vi "Error Query (Multiple).vi"(0 "VISA Resource Name":refnum<visa-resource-name>, 11 "error in (no error)":errorcluster {"code" format="%.0x"}) -> (4 "VISA Resource Name Out":refnum<visa-resource-name>, 8 "Error":i32[](array[numeric]), 10 "Error Message":string, 15 "error out":errorcluster {"code" format="%.0x"})   [LabVIEW 2012, in "Agilent ESG Series.lvlib"]
doc: "This VI reads the error queue from the instrument. It expects to see errors in SCPI format (#,\"error message\"). It continues to read from the error queue until it reads a 0, \"No error\". If the instrument does not support an error query, a warning is returned."
uses:
  <instrlib>/Agilent ESG Series/Agilent ESG Series.lvlib
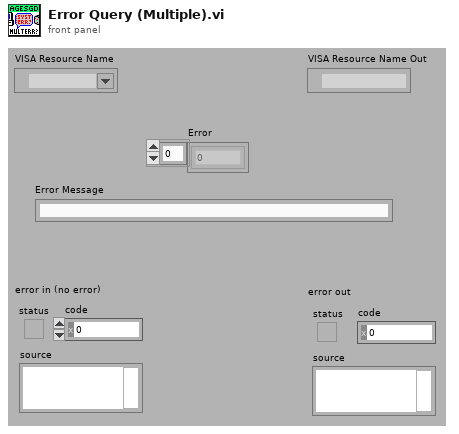
[diagram p1: front panel]
types:
  T1 = cluster{"Status":bool, "Error":i32, "source":string}
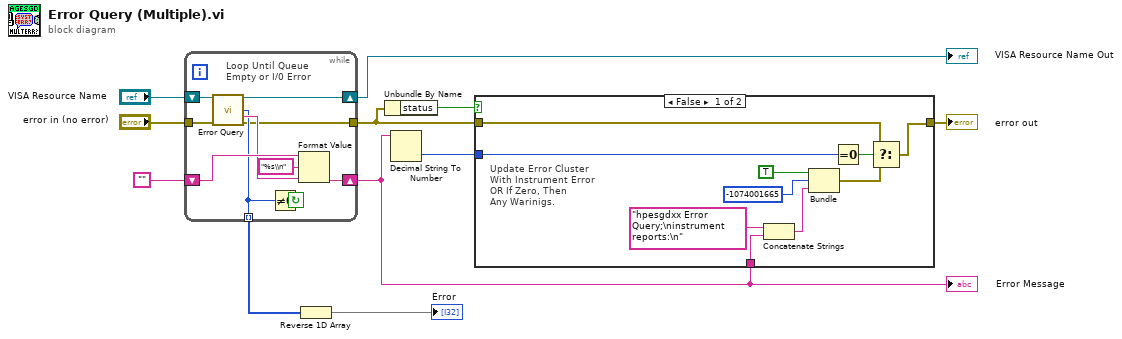
[diagram p0: block diagram]
diagram:
  n1 = while {
    tunnel: "error in (no error)" -> [w12]
    tunnel: [w15] -> w9 mode=indexing
    tunnel: [w13] -> w4
    shift-left: "VISA Resource Name" -> [w14]
    shift-right: [w21] -> w3
    shift-left: "" -> [w18]
    shift-right: [w20] -> w2
    stop <- w16 continue-if-true
    # "Loop Until Queue Empty or I/0 Error"
    n2 = call <instrlib>:"Error Query.vi"("VISA Resource Name"=w14, "error in (no error)"=w12) -> ("VISA Resource Name Out"=w21:refnum<visa-resource-name>, "Error"=w15:i32, "Error Message"=w17:string, "error out"=w13:errorcluster)  [unwired: 10 in]
    n3 = Not Equal To 0?(x=w15) -> (x != 0?=w16:bool)
    n4 = Format Value(string ("")=w18, format string="%s\\n", value (0)=w17) -> (output string=w20:string)
  }
  "Error Message" <- w2
  "VISA Resource Name Out" <- w3
  n5 = Reverse 1D Array(array=w9) -> (reversed array=→"Error":i32[])
  n6 = Unbundle By Name(w4) -> ("status"=w6:bool)
  n7 = Decimal String To Number(string=w2) -> (number=w5:i32)  [unwired: 2 in, 1 out]
  n8 = case shown="False" w6 {
    tunnel: w5 -> [w22 _]
    tunnel: [w25 w32] -> w7
    tunnel: w4 -> [w24 w32]
    tunnel: w2 -> [w31 _]
    frame False {
      # "Update Error Cluster\nWith Instrument Error \nOR If Zero, Then \nAny Warinigs."
      n9 = Concatenate Strings("hpesgdxx Error Query;\ninstrument reports:\n" ("Source"), w31) -> (w28:string)
      n10 = Bundle("Status"=TRUE, "Error"=-1074001665, w28) -> (w23:cluster{"Status":bool, "Error":i32, string})  [unwired: 1 in]
      n11 = Equal To 0?(x=w22) -> (x = 0?=w26:bool)
      n12 = Select(t=w24, s=w26, f=w23) -> (s? t:f=w25:T1)
    }
    frame True {
      # "IO Error"
    }
  }
  "error out" <- w7
